vi "Determine_tri_overlaps_PN.vi"(1 "Indices to check":i32[](array[numeric]), 2 "All triangles":T1[](array[typedef])) -> (0 "Max. no. of intersections":i32)   [LabVIEW 2011]
uses:
  Triangle2D.ctl
panel:
  # "Paul Nathan 04/03/10"
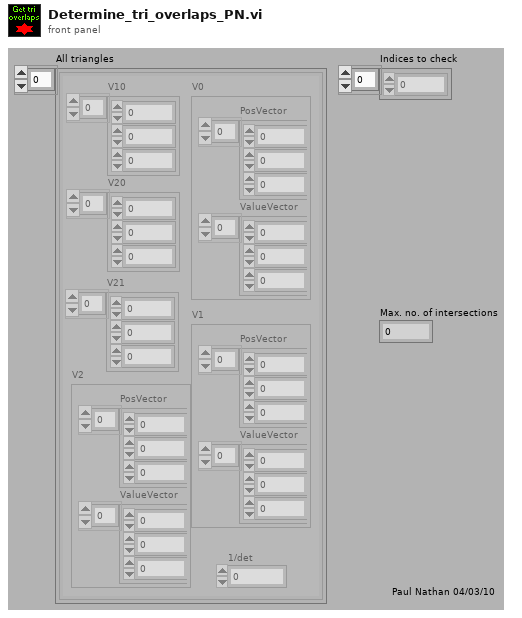
[diagram p1: front panel]
types:
  T1 = typedef "Triangle2D.ctl" = cluster{"V10":dbl[], "V20":dbl[], "1/det":dbl, "V0":cluster{"PosVector":dbl[], "ValueVector":dbl[]}, "V1":cluster{"PosVector":dbl[], "ValueVector":dbl[]}, "V2":cluster{"PosVector":dbl[], "ValueVector":dbl[]}, "V21":dbl[]}
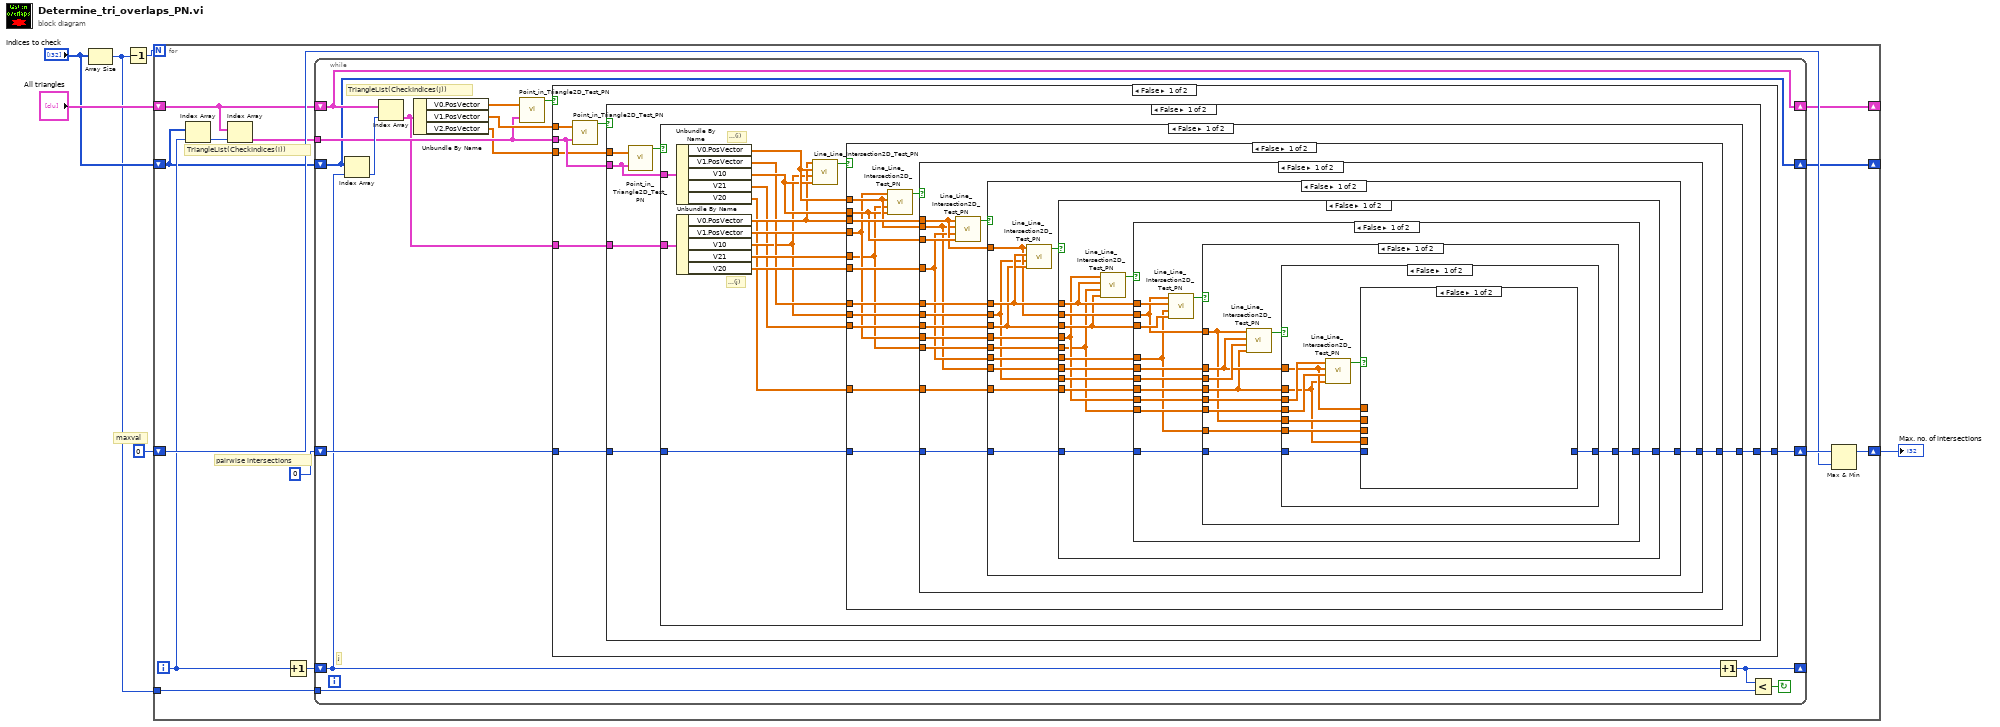
[diagram p0: block diagram]
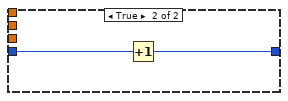
[diagram p2: hidden frame]
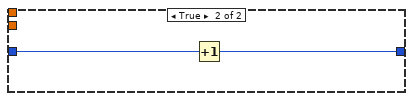
[diagram p3: hidden frame]
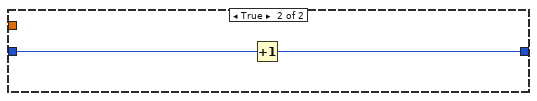
[diagram p4: hidden frame]
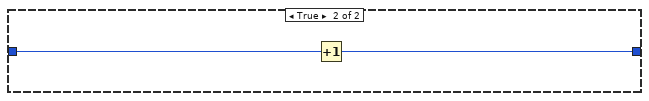
[diagram p5: hidden frame]
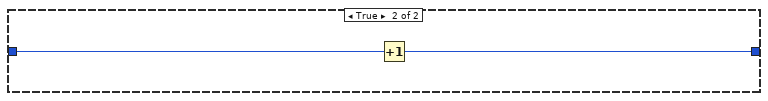
[diagram p6: hidden frame]
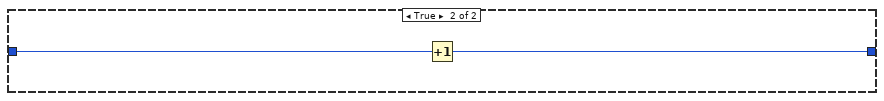
[diagram p7: hidden frame]
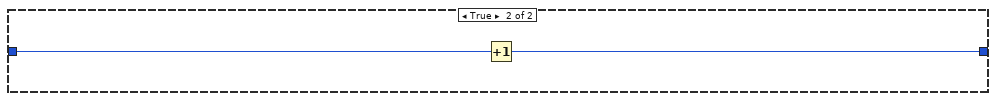
[diagram p8: hidden frame]
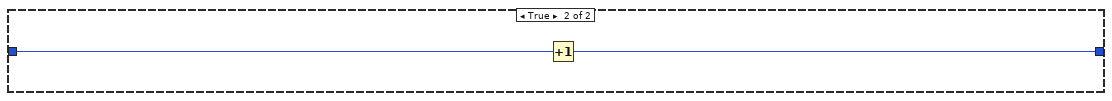
[diagram p9: hidden frame]
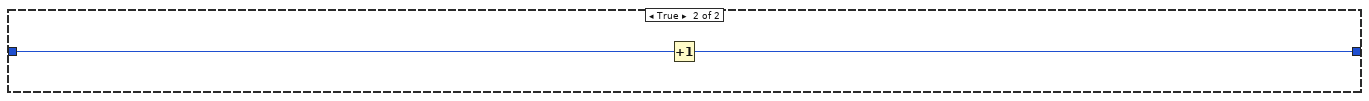
[diagram p10: hidden frame]
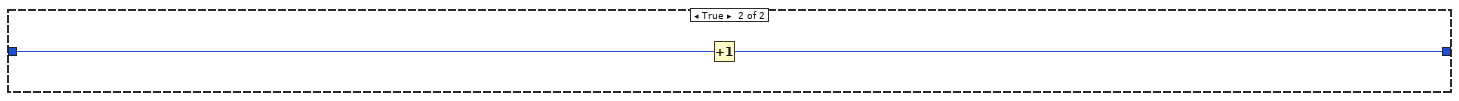
[diagram p11: hidden frame]
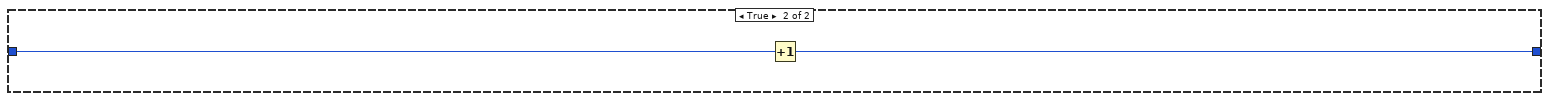
[diagram p12: hidden frame]
diagram:
  # "maxval"
  n1 = Array Size(array="Indices to check") -> (size(s)=w1:i32)
  n2 = Decrement(x=w1) -> (x-1=w6:i32)
  n3 = for {
    N: w6 -> [_]
    shift-right: [w15] -> w2
    shift-left: 0 -> [w16]
    tunnel: w1 -> [w9]
    shift-right: [w8] -> _
    shift-left: "All triangles" -> [w10]
    shift-right: [w7] -> _
    shift-left: "Indices to check" -> [w13]
    i -> [w14]
    # "pairwise intersections"
    # "TriangleList(CheckIndices(i))"
    n4 = Index Array(array=w13, index=w14) -> (element=w11:i32)
    n5 = Index Array(array=w10, index=w11) -> (element=w12:T1)
    n6 = Increment(x=w14) -> (x+1=w19:i32)
    n7 = while {
      tunnel: w9 -> [w34]
      shift-right: [w22] -> _
      shift-left: w19 -> [w23]
      shift-right: [w28] -> w17
      shift-left: 0 -> [w29]
      tunnel: w12 -> [w26]
      shift-right: [w21] -> w8
      shift-left: w10 -> [w21]
      shift-right: [w20] -> w7
      shift-left: w13 -> [w20]
      stop <- w33 continue-if-true
      # "j"
      # "TriangleList(CheckIndices(j))"
      n8 = Index Array(array=w20, index=w23) -> (element=w32:i32)
      n9 = Index Array(array=w21, index=w32) -> (element=w24:T1)
      n10 = Unbundle By Name(w24) -> ("V0.PosVector"=w31:dbl[], "V1.PosVector"=w27:dbl[], "V2.PosVector"=w25:dbl[])
      n11 = call "Point_in_Triangle2D_Test_PN.vi"("2D Point to Test"=w31, "Triangle2D"=w26) -> ("Point is in triangle"=w30:bool)  [unwired: 3 out]
      n12 = case shown="False" w30 {
        tunnel: w29 -> [w39 w175]
        tunnel: [w38 w174] -> w28
        tunnel: w27 -> [w41 _]
        tunnel: w26 -> [w37 _]
        tunnel: w25 -> [w36 _]
        tunnel: w24 -> [w35 _]
        frame False {
          n13 = call "Point_in_Triangle2D_Test_PN.vi"("2D Point to Test"=w41, "Triangle2D"=w37) -> ("Point is in triangle"=w40:bool)  [unwired: 3 out]
          n14 = case shown="False" w40 {
            tunnel: w39 -> [w45 w173]
            tunnel: [w44 w172] -> w38
            tunnel: w37 -> [w43 _]
            tunnel: w36 -> [w47 _]
            tunnel: w35 -> [w42 _]
            frame False {
              n15 = call "Point_in_Triangle2D_Test_PN.vi"("2D Point to Test"=w47, "Triangle2D"=w43) -> ("Point is in triangle"=w46:bool)  [unwired: 3 out]
              n16 = case shown="False" w46 {
                tunnel: w45 -> [w59 w171]
                tunnel: [w58 w170] -> w44
                tunnel: w43 -> [w62 _]
                tunnel: w42 -> [w61 _]
                frame False {
                  # "...(j)"
                  # "...(i)"
                  n17 = Unbundle By Name(w62) -> ("V0.PosVector"=w57:dbl[], "V1.PosVector"=w51:dbl[], "V10"=w56:dbl[], "V21"=w49:dbl[], "V20"=w48:dbl[])
                  n18 = Unbundle By Name(w61) -> ("V0.PosVector"=w53:dbl[], "V1.PosVector"=w55:dbl[], "V10"=w50:dbl[], "V21"=w54:dbl[], "V20"=w52:dbl[])
                  n19 = call "Line_Line_Intersection2D_Test_PN.vi"("2D Dir. Vect. of Line 2 (not unit)"=w56, "2D Dir. Vect. of Line 1 (not unit)"=w50, "2D Point on Line 2"=w57, "2D Point on Line 1"=w53) -> ("Lines Intersect"=w60:bool)  [unwired: 2 out]
                  n20 = case shown="False" w60 {
                    tunnel: w59 -> [w74 w169]
                    tunnel: [w73 w168] -> w58
                    tunnel: w57 -> [w71 _]
                    tunnel: w56 -> [w70 _]
                    tunnel: w55 -> [w65 _]
                    tunnel: w54 -> [w64 _]
                    tunnel: w53 -> [w72 _]
                    tunnel: w52 -> [w69 _]
                    tunnel: w51 -> [w68 _]
                    tunnel: w50 -> [w67 _]
                    tunnel: w49 -> [w66 _]
                    tunnel: w48 -> [w63 _]
                    frame False {
                      n21 = call "Line_Line_Intersection2D_Test_PN.vi"("2D Dir. Vect. of Line 2 (not unit)"=w70, "2D Dir. Vect. of Line 1 (not unit)"=w64, "2D Point on Line 2"=w71, "2D Point on Line 1"=w65) -> ("Lines Intersect"=w75:bool)  [unwired: 2 out]
                      n22 = case shown="False" w75 {
                        tunnel: w74 -> [w86 w167]
                        tunnel: [w85 w166] -> w73
                        tunnel: w72 -> [w84 _]
                        tunnel: w71 -> [w77 _]
                        tunnel: w70 -> [w88 _]
                        tunnel: w69 -> [w78 _]
                        tunnel: w68 -> [w83 _]
                        tunnel: w67 -> [w82 _]
                        tunnel: w66 -> [w81 _]
                        tunnel: w65 -> [w80 _]
                        tunnel: w64 -> [w79 _]
                        tunnel: w63 -> [w76 _]
                        frame False {
                          n23 = call "Line_Line_Intersection2D_Test_PN.vi"("2D Dir. Vect. of Line 2 (not unit)"=w88, "2D Dir. Vect. of Line 1 (not unit)"=w78, "2D Point on Line 2"=w77, "2D Point on Line 1"=w84) -> ("Lines Intersect"=w87:bool)  [unwired: 2 out]
                          n24 = case shown="False" w87 {
                            tunnel: w86 -> [w99 w165]
                            tunnel: [w98 w164] -> w85
                            tunnel: w84 -> [w93 _]
                            tunnel: w83 -> [w96 _]
                            tunnel: w82 -> [w90 _]
                            tunnel: w81 -> [w94 _]
                            tunnel: w80 -> [w97 _]
                            tunnel: w79 -> [w95 _]
                            tunnel: w78 -> [w92 _]
                            tunnel: w77 -> [w91 _]
                            tunnel: w76 -> [w89 _]
                            frame False {
                              n25 = call "Line_Line_Intersection2D_Test_PN.vi"("2D Dir. Vect. of Line 2 (not unit)"=w94, "2D Dir. Vect. of Line 1 (not unit)"=w90, "2D Point on Line 2"=w96, "2D Point on Line 1"=w93) -> ("Lines Intersect"=w100:bool)  [unwired: 2 out]
                              n26 = case shown="False" w100 {
                                tunnel: w99 -> [w110 w163]
                                tunnel: [w111 w162] -> w98
                                tunnel: w97 -> [w102 _]
                                tunnel: w96 -> [w108 _]
                                tunnel: w95 -> [w101 _]
                                tunnel: w94 -> [w106 _]
                                tunnel: w93 -> [w109 _]
                                tunnel: w92 -> [w107 _]
                                tunnel: w91 -> [w105 _]
                                tunnel: w90 -> [w104 _]
                                tunnel: w89 -> [w103 _]
                                frame False {
                                n27 = call "Line_Line_Intersection2D_Test_PN.vi"("2D Dir. Vect. of Line 2 (not unit)"=w106, "2D Dir. Vect. of Line 1 (not unit)"=w101, "2D Point on Line 2"=w108, "2D Point on Line 1"=w102) -> ("Lines Intersect"=w112:bool)  [unwired: 2 out]
                                n28 = case shown="False" w112 {
                                tunnel: [w120 w161] -> w111
                                tunnel: w110 -> [w121 w160]
                                tunnel: w109 -> [w119 _]
                                tunnel: w108 -> [w124 _]
                                tunnel: w107 -> [w113 _]
                                tunnel: w106 -> [w123 _]
                                tunnel: w105 -> [w118 _]
                                tunnel: w104 -> [w117 _]
                                tunnel: w103 -> [w116 _]
                                tunnel: w102 -> [w115 _]
                                tunnel: w101 -> [w114 _]
                                frame False {
                                n29 = call "Line_Line_Intersection2D_Test_PN.vi"("2D Dir. Vect. of Line 2 (not unit)"=w123, "2D Dir. Vect. of Line 1 (not unit)"=w113, "2D Point on Line 2"=w124, "2D Point on Line 1"=w119) -> ("Lines Intersect"=w122:bool)  [unwired: 2 out]
                                n30 = case shown="False" w122 {
                                tunnel: w121 -> [w132 w159]
                                tunnel: [w131 w158] -> w120
                                tunnel: w119 -> [w126 _]
                                tunnel: w118 -> [w129 _]
                                tunnel: w117 -> [w134 _]
                                tunnel: w116 -> [w127 _]
                                tunnel: w115 -> [w130 _]
                                tunnel: w114 -> [w128 _]
                                tunnel: w113 -> [w125 _]
                                frame False {
                                n31 = call "Line_Line_Intersection2D_Test_PN.vi"("2D Dir. Vect. of Line 2 (not unit)"=w127, "2D Dir. Vect. of Line 1 (not unit)"=w134, "2D Point on Line 2"=w129, "2D Point on Line 1"=w126) -> ("Lines Intersect"=w133:bool)  [unwired: 2 out]
                                n32 = case shown="False" w133 {
                                tunnel: w132 -> [w141 w157]
                                tunnel: [w140 w156] -> w131
                                tunnel: w130 -> [w143 _]
                                tunnel: w129 -> [w137 _]
                                tunnel: w128 -> [w142 _]
                                tunnel: w127 -> [w135 _]
                                tunnel: w126 -> [w139 _]
                                tunnel: w125 -> [w136 _]
                                frame False {
                                n33 = call "Line_Line_Intersection2D_Test_PN.vi"("2D Dir. Vect. of Line 2 (not unit)"=w135, "2D Dir. Vect. of Line 1 (not unit)"=w142, "2D Point on Line 2"=w137, "2D Point on Line 1"=w143) -> ("Lines Intersect"=w138:bool)  [unwired: 2 out]
                                n34 = case shown="False" w138 {
                                tunnel: w141 -> [w145 w155]
                                tunnel: [w144 w154] -> w140
                                tunnel: w139 -> [w150 _]
                                tunnel: w137 -> [w149 _]
                                tunnel: w136 -> [w148 _]
                                tunnel: w135 -> [w147 _]
                                frame False {
                                n35 = call "Line_Line_Intersection2D_Test_PN.vi"("2D Dir. Vect. of Line 2 (not unit)"=w147, "2D Dir. Vect. of Line 1 (not unit)"=w148, "2D Point on Line 2"=w149, "2D Point on Line 1"=w150) -> ("Lines Intersect"=w146:bool)  [unwired: 2 out]
                                n36 = case shown="True" w146 {
                                tunnel: w145 -> [w151 w153]
                                tunnel: [w151 w152] -> w144
                                frame False {
                                }
                                frame True {
                                n37 = Increment(x=w153) -> (x+1=w152:i32)
                                }
                                }
                                }
                                frame True {
                                n38 = Increment(x=w155) -> (x+1=w154:i32)
                                }
                                }
                                }
                                frame True {
                                n39 = Increment(x=w157) -> (x+1=w156:i32)
                                }
                                }
                                }
                                frame True {
                                n40 = Increment(x=w159) -> (x+1=w158:i32)
                                }
                                }
                                }
                                frame True {
                                n41 = Increment(x=w160) -> (x+1=w161:i32)
                                }
                                }
                                }
                                frame True {
                                n42 = Increment(x=w163) -> (x+1=w162:i32)
                                }
                              }
                            }
                            frame True {
                              n43 = Increment(x=w165) -> (x+1=w164:i32)
                            }
                          }
                        }
                        frame True {
                          n44 = Increment(x=w167) -> (x+1=w166:i32)
                        }
                      }
                    }
                    frame True {
                      n45 = Increment(x=w169) -> (x+1=w168:i32)
                    }
                  }
                }
                frame True {
                  n46 = Increment(x=w171) -> (x+1=w170:i32)
                }
              }
            }
            frame True {
              n47 = Increment(x=w173) -> (x+1=w172:i32)
            }
          }
        }
        frame True {
          n48 = Increment(x=w175) -> (x+1=w174:i32)
        }
      }
      n49 = Increment(x=w23) -> (x+1=w22:i32)
      n50 = Less?(x=w22, y=w34) -> (x < y?=w33:bool)
    }
    n51 = Max & Min(x=w17, y=w16) -> (max(x,y)=w15:i32)  [unwired: 1 out]
  }
  "Max. no. of intersections" <- w2
